vi "streamWrite.vi"(8 "error in (no error)":errorcluster, 10 "String":string, 11 "TestTestResult in":refnum<class "_TextTestResult.lvclass">) -> (0 "error out":errorcluster, 3 "TestTestResult out":refnum<class "_TextTestResult.lvclass">)   [LabVIEW 2011, in "_TextTestResult.lvclass"]
uses:
  _TextTestResult.lvclass
  _TextTestResult.lvclass/_TextTestResult.ctl
panel:
  # "JKI VI Tester for LabVIEW\nhttp://jkisoft.com/vi-tester\nCopyright (C) 2007-2009, JKI <info@jkisoft.com>\nALL RIGHTS RESERVED"
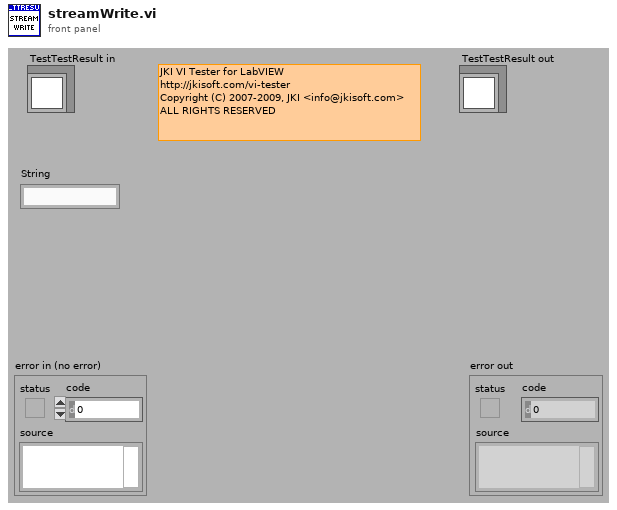
[diagram p1: front panel]
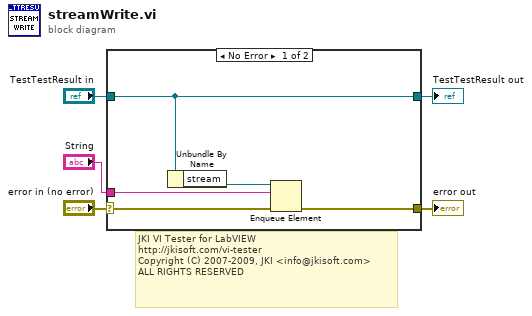
[diagram p0: block diagram]
diagram:
  # "JKI VI Tester for LabVIEW\nhttp://jkisoft.com/vi-tester\nCopyright (C) 2007-2009, JKI <info@jkisoft.com>\nALL RIGHTS RESERVED"
  n1 = case shown="No Error" "error in (no error)" {
    selector: "error in (no error)" -> [w8 w12]
    tunnel: [w7 w12] -> w4
    tunnel: [w10 w11] -> w2
    tunnel: "TestTestResult in" -> [w10 w11]
    tunnel: "String" -> [w6 _]
    frame No Error {
      n2 = Unbundle By Name(w10) -> ("stream"=w9:refnum<queue>)
      n3 = Enqueue Element(queue=w9, element=w6, error in (no error)=w8) -> (error out=w7:errorcluster)  [unwired: 1 in, 2 out]
    }
    frame Error {
    }
  }
  "error out" <- w4
  "TestTestResult out" <- w2
